vi "FTW-ERR-Explanation.vi"(1 "error to check":errorcluster) -> (0 "Explanation":string)   [LabVIEW 2014]
panel:
  # "Inputs"
  # "Outputs"
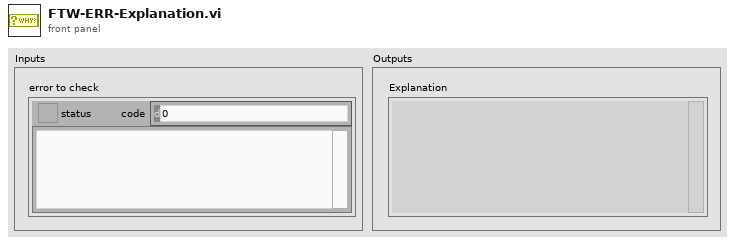
[diagram p1: front panel]
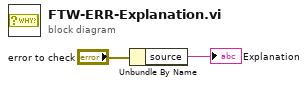
[diagram p0: block diagram]
diagram:
  n1 = Unbundle By Name("error to check") -> ("source"=→"Explanation":string)
